vi "ConfigureOVA.vi"(4 "error in":errorcluster, 6 "VIS?":bool, 7 "Use INI File?":bool) -> (0 "error out":errorcluster, 1 "memError":bool, 2 "Cfg OK?":bool, 3 "instrFound":bool)   [LabVIEW 2024]
uses:
  OVA32.dll
panel:
  # "Configure OVA"
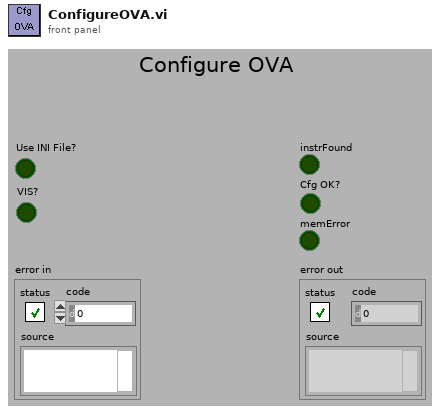
[diagram p1: front panel]
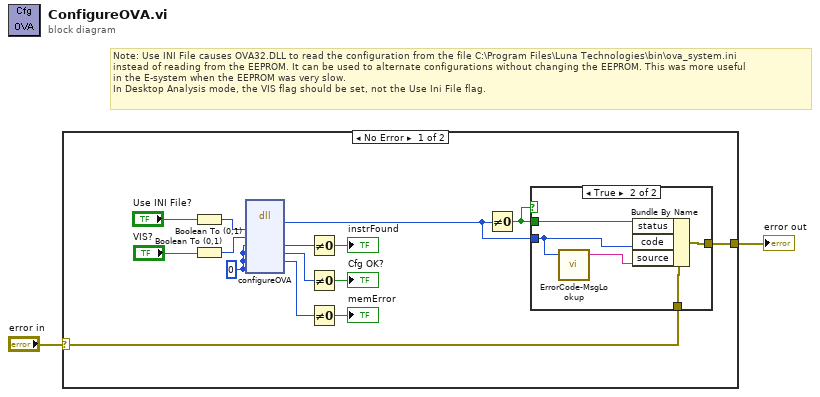
[diagram p0: block diagram]
diagram:
  # "Note: Use INI File causes OVA32.DLL to read the configuration from the file C:\\Program Files\\Luna Technologies\\bin\\ova_system.ini\ninstead of reading from the EEPROM. It can be used to alternate configurations without changing the EEPROM. This was more useful\nin the E-system when the EEPROM was very slow.\nIn Desktop Analysis mode, the VIS flag should be set, not the Use Ini File flag."
  n1 = case shown="No Error" "error in" {
    selector: "error in" -> [w6 w24]
    tunnel: [w7 w24] -> w2
    frame No Error {
      w16 = u8 0 ("instrFound")
      n2 = Boolean To (0,1)(Boolean="Use INI File?") -> (0, 1=w5:i16)
      n3 = Boolean To (0,1)(Boolean="VIS?") -> (0, 1=w3:i16)
      n4 = dll-call lib="OVA32.dll" fn="configureOVA"("loadFromFile"=w5, "vis"=w3, "instrFound"=w16, "configOK"=w16, "memError"=w16, "numMatrices"=w16) -> ("return type"=w8:i32, "instrFound"=w15:u8, "configOK"=w13:u8, "memError"=w11:u8)  [unwired: 6 in, 2 out]
      n5 = Not Equal To 0?(x=w15) -> (x != 0?=→"instrFound":bool)
      n6 = Not Equal To 0?(x=w13) -> (x != 0?=→"Cfg OK?":bool)
      n7 = Not Equal To 0?(x=w11) -> (x != 0?=→"memError":bool)
      n8 = Not Equal To 0?(x=w8) -> (x != 0?=w9:bool)
      n9 = case shown="True" w9 {
        tunnel: w9 -> [_ w23]
        tunnel: [w18 w22] -> w7
        tunnel: w8 -> [_ w21]
        tunnel: w6 -> [w18 w19]
        frame False {
        }
        frame True {
          n10 = call "ErrorCode-MsgLookup.vi"("DLL Return Code"=w21) -> ("Error String"=w20:string)  [unwired: 2 in, 2 out]
          n11 = Bundle By Name(cluster=w19, "status"=w23, "code"=w21, "source"=w20) -> (w22:errorcluster)
        }
      }
    }
    frame Error {
    }
  }
  "error out" <- w2
